vi "Read CPU Temps.vi"(8 "error in (no error)":errorcluster) -> (0 "error out":errorcluster, 2 "Termperatures":dbl[](array[numeric]), 3 "Names":string[](array[string]))   [LabVIEW 2020]
uses:
  C:/Users/Josh/Desktop/code/sandbox/ni/read_temp/OpenHardwareMonitorLib.dll
  OpenHardwareMonitorLib.dll
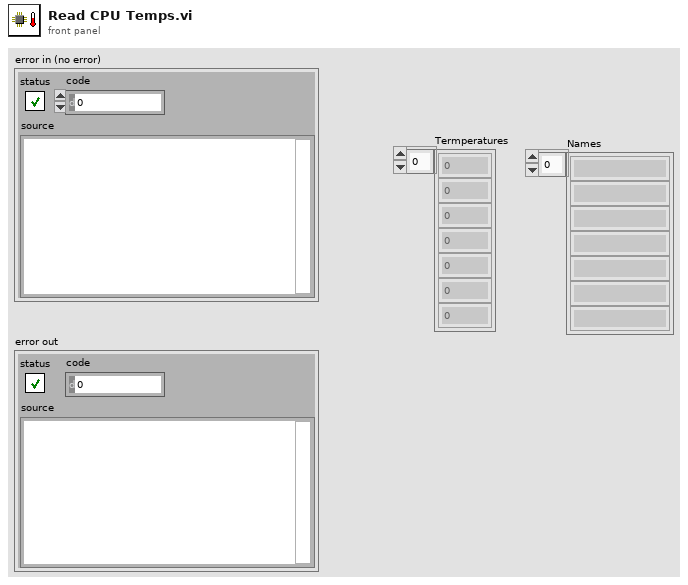
[diagram p1: front panel]
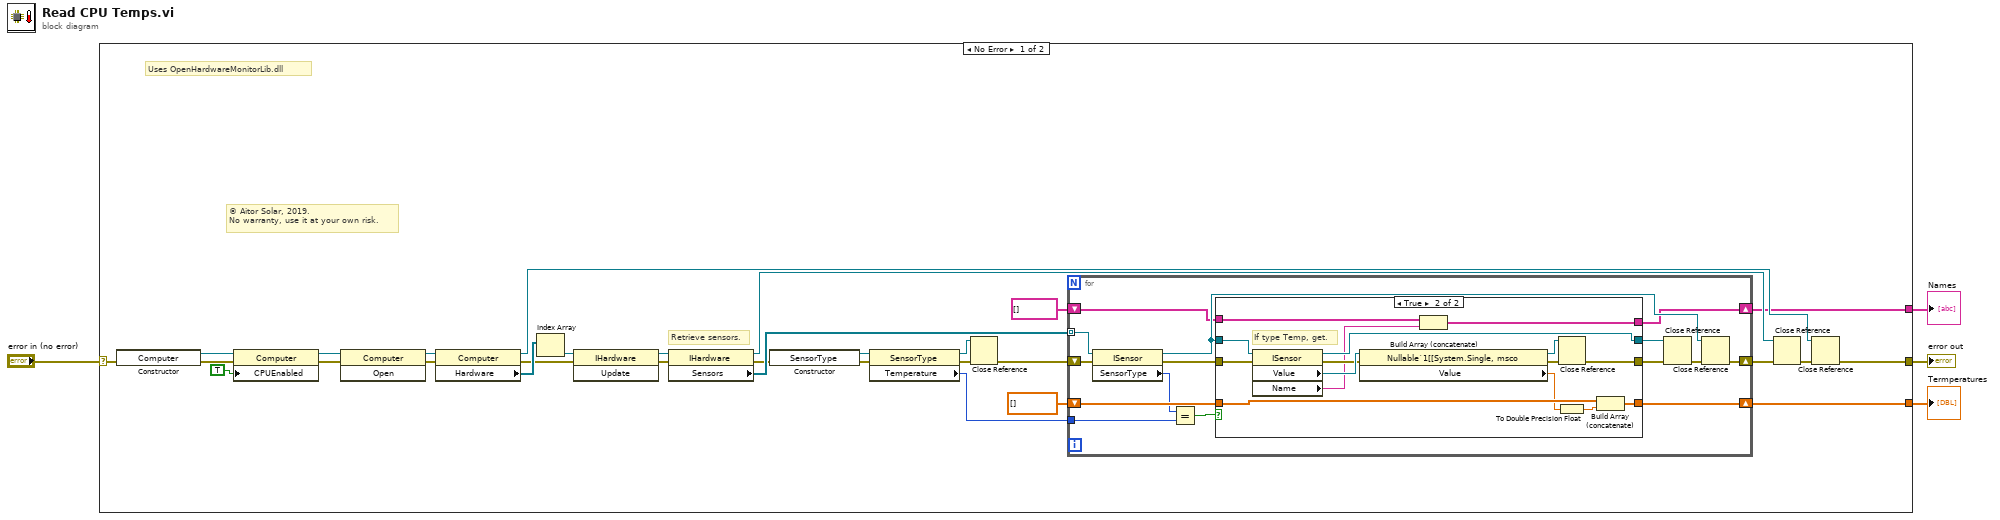
[diagram p0: block diagram]
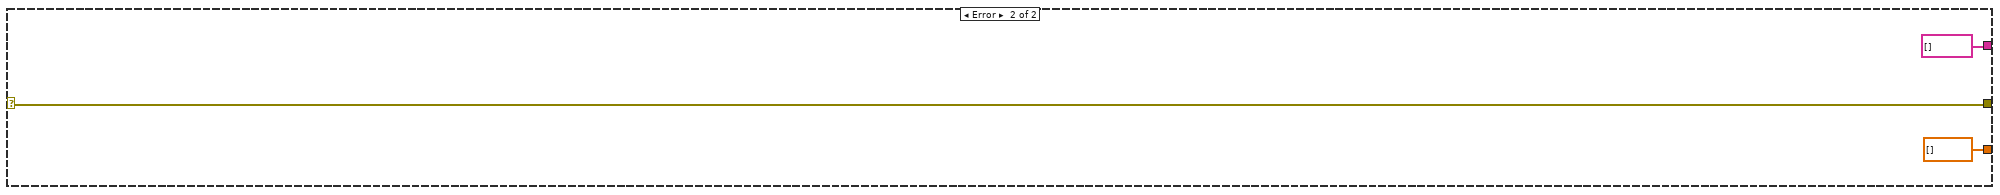
[diagram p3: hidden frame]
diagram:
  n1 = case shown="No Error" "error in (no error)" {
    selector: "error in (no error)" -> [w17 w71]
    tunnel: [w18 w71] -> w3
    tunnel: [w7 dbl[] []] -> w2
    tunnel: [w5 string[] []] -> w1
    frame No Error {
      # "© Aitor Solar, 2019.\nNo warranty, use it at your own risk."
      # "Uses OpenHardwareMonitorLib.dll"
      # "Retrieve sensors."
      n2 = constructor class="Computer"(error in=w17) -> (reference out=w11:refnum<k24>, error out=w16:errorcluster)  [unwired: 2 in, 1 out]
      n3 = property class="Computer"(reference=w11, error in=w16, "CPUEnabled"=TRUE) -> (reference out=w12:refnum<k24>, error out=w15:errorcluster)
      n4 = invoke class="Computer" method="Open"(reference=w12, error in=w15) -> (reference out=w13:refnum<k24>, error out=w14:errorcluster)  [unwired: 1 in, 1 out]
      n5 = property class="Computer"(reference=w13, error in=w14) -> (reference out=w19:refnum<k24>, error out=w29:errorcluster, "Hardware"=w34:refnum<k24>[])
      n6 = Index Array(array=w34) -> (element=w31:refnum<k24>)  [unwired: 1 in]
      n7 = invoke class="IHardware" method="Update"(reference=w31, error in=w29) -> (reference out=w30:refnum<k24>, error out=w28:errorcluster)  [unwired: 1 in, 1 out]
      n8 = property class="IHardware"(reference=w30, error in=w28) -> (reference out=w21:refnum<k24>, error out=w25:errorcluster, "Sensors"=w32:refnum<k24>[])
      n9 = constructor class="SensorType"(error in=w25) -> (reference out=w26:refnum<k24>, error out=w27:errorcluster)  [unwired: 2 in, 1 out]
      n10 = property class="SensorType"(reference=w26, error in=w27) -> (reference out=w22:refnum<k24>, error out=w9:errorcluster, "Temperature"=w24:i32)
      n11 = Close Reference(reference=w22, error in (no error)=w9) -> (error out=w8:errorcluster)
      n12 = for {
        tunnel: w32 -> [w48] mode=indexing
        shift-right: [w40] -> w10
        shift-left: w8 -> [w47]
        tunnel: w24 -> [w45]
        shift-right: [w49] -> w7
        shift-left: dbl[] [] -> [w43]
        shift-right: [w35] -> w5
        shift-left: string[] [] -> [w36]
        n13 = property class="ISensor"(reference=w48, error in=w47) -> (reference out=w37:refnum<k24>, error out=w46:errorcluster, "SensorType"=w38:i32)
        n14 = Equal?(x=w38, y=w45) -> (x = y?=w44:bool)
        n15 = case shown="True" w44 {
          tunnel: [w53 w67] -> w49
          tunnel: w46 -> [w52 w65]
          tunnel: w43 -> [w53 w68]
          tunnel: [w52 w58] -> w42
          tunnel: [w51 w63] -> w41
          tunnel: w37 -> [w51 w64]
          tunnel: w36 -> [w50 w55]
          tunnel: [w50 w54] -> w35
          frame False {
          }
          frame True {
            # "If type Temp, get."
            n16 = property class="ISensor"(reference=w64, error in=w65) -> (reference out=w63:refnum<k24>, error out=w57:errorcluster, "Value"=w62:refnum<k24>, "Name"=w56:string)
            n17 = property class="Nullable`1[[System.Single, msco"(reference=w62, error in=w57) -> (reference out=w60:refnum<k24>, error out=w59:errorcluster, "Value"=w61:sgl)
            n18 = Build Array (concatenate)(w55, w56) -> (w54:string[])
            n19 = Close Reference(reference=w60, error in (no error)=w59) -> (error out=w58:errorcluster)
            n20 = To Double Precision Float(number=w61) -> (double precision float=w66:dbl)
            n21 = Build Array (concatenate)(w68, w66) -> (w67:dbl[])
          }
        }
        n22 = Close Reference(reference=w41, error in (no error)=w42) -> (error out=w39:errorcluster)
        n23 = Close Reference(reference=w37, error in (no error)=w39) -> (error out=w40:errorcluster)
      }
      n24 = Close Reference(reference=w21, error in (no error)=w10) -> (error out=w20:errorcluster)
      n25 = Close Reference(reference=w19, error in (no error)=w20) -> (error out=w18:errorcluster)
    }
    frame Error {
    }
  }
  "error out" <- w3
  "Termperatures" <- w2
  "Names" <- w1
